vi "Jog XY go.vi"(9 "Speed":dbl=5.0, 10 "Jog Cluster IN":T1={"Jog XY Cluster"={"object goes up"=FALSE, "object goes down"=FALSE, "object goes right"=FALSE, "object goes left"=FALSE, "SW2"=FALSE, "SW1"=FALSE, "YY (mm)"=0.1, "YN (mm) "=0.01, "NY (mm) "=0.005, "NN (mm) "=0.001}, "Jog Z Cluster "={"Z go down 0.1 mm"=FALSE, "Z go up 0.1 mm"=FALSE, "Z go down 0.05 mm"=FALSE, "Z go up 0.05 mm"=FALSE, "Z go down 0.01 mm"=FALSE, "Z go up 0.01 mm"=FALSE, "Z go down"=FALSE, "Z go up"=FALSE, "step (mm)"=0.001}}, 11 "Motion.lvclass IN":refnum<class "Motion.lvclass">) -> (2 "Jog Cluster OUT":T1={"Jog XY Cluster"={"object goes up"=FALSE, "object goes down"=FALSE, "object goes right"=FALSE, "object goes left"=FALSE, "SW2"=FALSE, "SW1"=FALSE, "YY (mm)"=0.1, "YN (mm) "=0.01, "NY (mm) "=0.005, "NN (mm) "=0.001}, "Jog Z Cluster "={"Z go down 0.1 mm"=FALSE, "Z go up 0.1 mm"=FALSE, "Z go down 0.05 mm"=FALSE, "Z go up 0.05 mm"=FALSE, "Z go down 0.01 mm"=FALSE, "Z go up 0.01 mm"=FALSE, "Z go down"=FALSE, "Z go up"=FALSE, "step (mm)"=0.001}}, 3 "Motion.lvclass OUT":refnum<class "Motion.lvclass">)   [LabVIEW 2016]
uses:
  Classes/Controller/Motion/Motion.lvclass
panel:
  in  "Tab Control":enum32{"jog", "controller"}(tab)
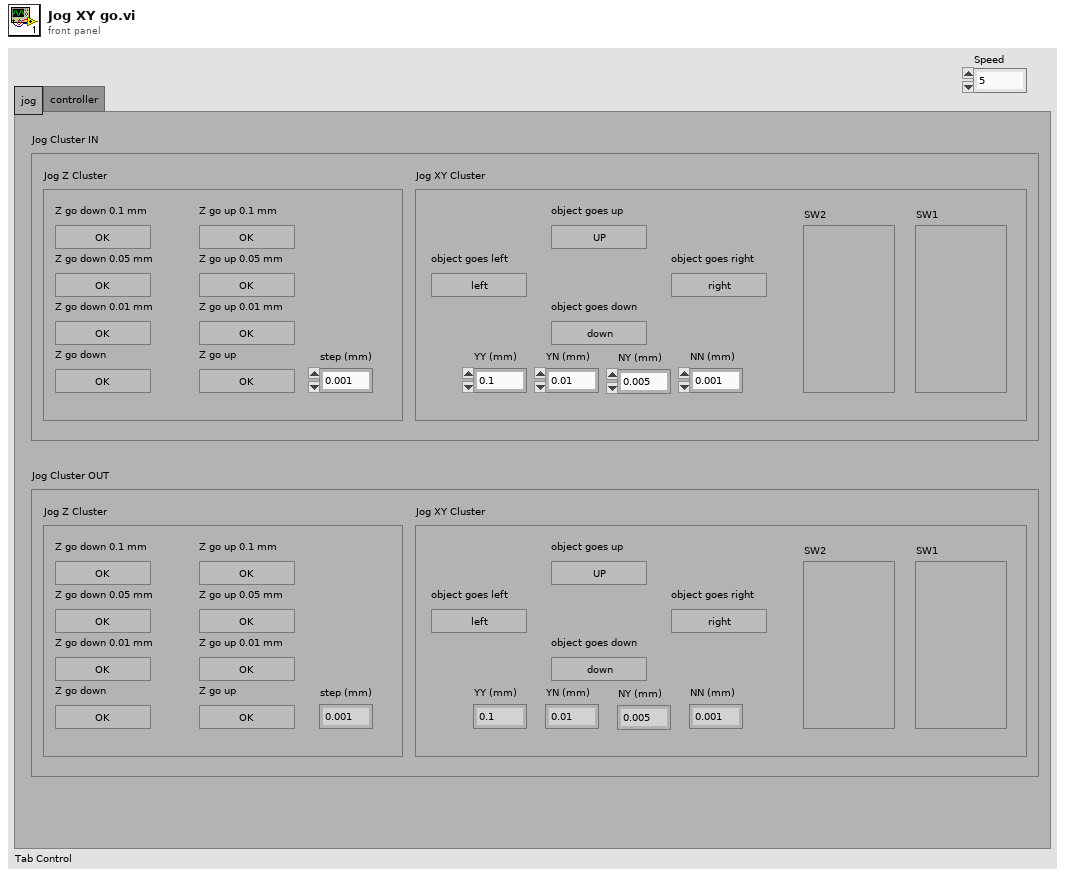
[diagram p1: front panel]
types:
  T1 = cluster{"Jog XY Cluster":cluster{"object goes up":bool, "object goes down":bool, "object goes right":bool, "object goes left":bool, "SW2":bool, "SW1":bool, "YY (mm)":dbl, "YN (mm) ":dbl, "NY (mm) ":dbl, "NN (mm) ":dbl}, "Jog Z Cluster ":cluster{"Z go down 0.1 mm":bool, "Z go up 0.1 mm":bool, "Z go down 0.05 mm":bool, "Z go up 0.05 mm":bool, "Z go down 0.01 mm":bool, "Z go up 0.01 mm":bool, "Z go down":bool, "Z go up":bool, "step (mm)":dbl}}
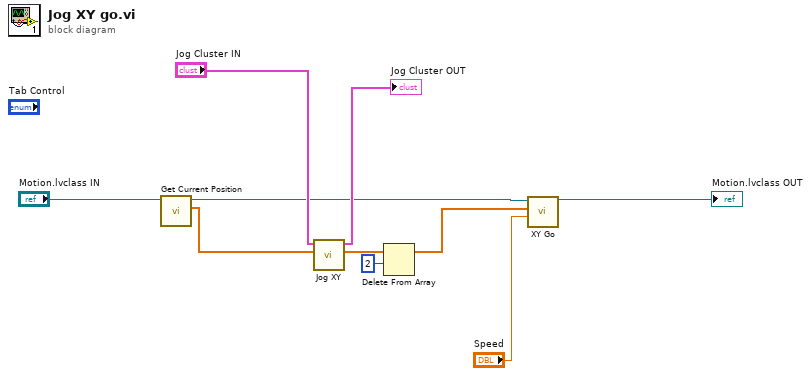
[diagram p0: block diagram]
diagram:
  n1 = call-dynamic "Get Current Position.vi"("Motion in"="Motion.lvclass IN") -> ("XYZTheta Out"=w7:dbl[], "Motion out"=w5:refnum<class "Motion.lvclass">)  [unwired: 8 in, 1 out]
  n2 = call "Jog XY.vi"("array IN"=w7, "Jog Cluster"="Jog Cluster IN") -> ("array OUT"=w2:dbl[], "Jog Cluster output"=→"Jog Cluster OUT":T1)  [unwired: 8 in]
  n3 = Delete From Array(array=w2, length=2) -> (array with subset deleted=w1:dbl[])  [unwired: 1 in, 1 out]
  n4 = call-dynamic "XY Go.vi"("Speed"="Speed", "XY"=w1, "Motion in"=w5) -> ("Motion out"=→"Motion.lvclass OUT":refnum<class "Motion.lvclass">)  [unwired: 7 in, 1 out]
